vi "Assert No Error.vi"(7 "Status":T1=enum."Failed", 8 "error In":errorcluster, 10 "Assert error":errorcluster, 11 "LUnit Test Case In":refnum<class "LUnit Test Case V2.lvclass">) -> (0 "error out":errorcluster, 3 "LUnit Test Case Out":refnum<class "LUnit Test Case V2.lvclass">)   [LabVIEW 2020, in "LUnit Test Case V2.lvclass"]
doc: "Generates a fail result for the calling test method if the inputs contains an error with status \"True\". A description may be provided to the result."
uses:
  LUnit Test Case V2.lvclass
  Result/Status.ctl
  Result/Type.ctl
  Result/Result.ctl
  LUnit Test Case V2.lvclass/LUnit Test Case V2.ctl
  Result/Result.lvlib
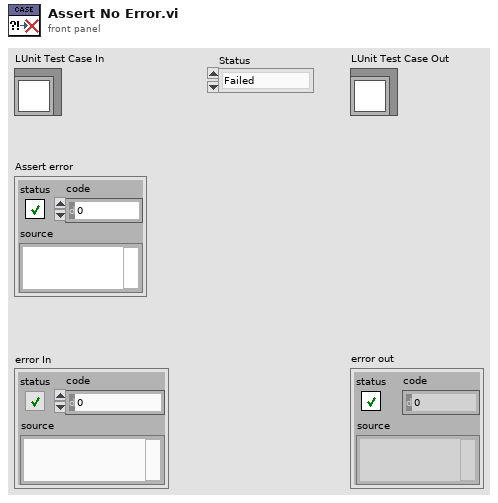
[diagram p1: front panel]
types:
  T1 = typedef "Result.lvlib/Status.ctl" = enum16{"", "Passed", "Failed", "Error", "Skipped", "Setup Error", "Broken", "Teardown Error"}
  T2 = typedef "Result.lvlib/Type.ctl" = enum16{"Method", "Case", "Suite", "Pass", "Fail", "Skip", "Pass if", "Fail if", "Pass if Error", "Fail if Error", "Pass if Equal", "Fail if Equal"}
  T3 = typedef "Result.lvlib/Result.ctl" = cluster{"Name":string, "Message":string, "Description":string, "Status":T1, "Result Type":T2, "Execution Time":dbl}
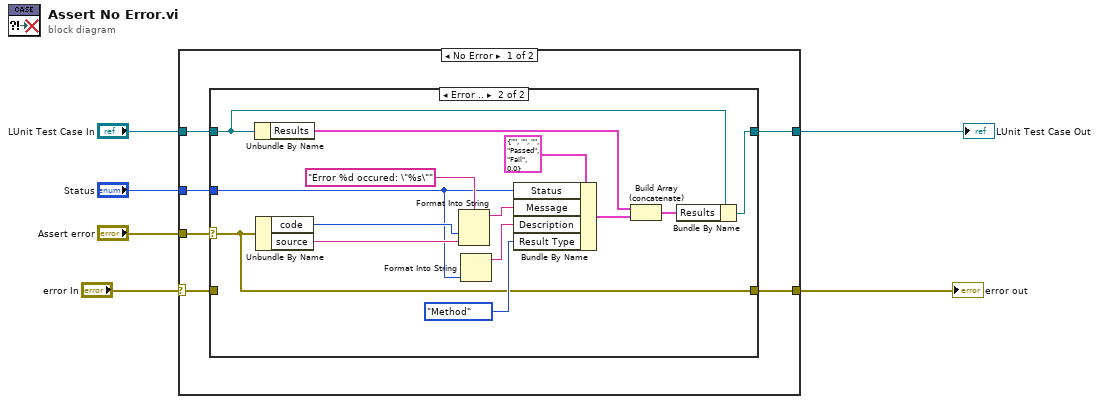
[diagram p0: block diagram]
diagram:
  n1 = case shown="No Error" "error In" {
    selector: "error In" -> [w7 w30]
    tunnel: "Assert error" -> [w12 _]
    tunnel: "LUnit Test Case In" -> [w11 w29]
    tunnel: [w10 w29] -> w4
    tunnel: "Status" -> [w9 _]
    tunnel: [w8 w30] -> w2
    frame No Error {
      n2 = case shown="Error .." w12 {
        selector: w12 -> [_ w15]
        tunnel: w11 -> [w14 w28]
        tunnel: [w14 w27] -> w10
        tunnel: w9 -> [_ w17]
        tunnel: [w13 w15] -> w8
        tunnel: w7 -> [w13 _]
        frame No Error {
        }
        frame Error {
          n3 = Unbundle By Name(w28) -> ("Results"=w21:T3[])
          n4 = Unbundle By Name(w15) -> ("code"=w24:i32, "source"=w23:string)
          n5 = Format Into String(format string="Error %d occured: \"%s\"", w24, w23) -> (resulting string=w26:string)  [unwired: 2 in, 1 out]
          n6 = Format Into String(w17) -> (resulting string=w16:string)  [unwired: 3 in, 1 out]
          n7 = Bundle By Name(cluster=T3 {"Name"="", "Message"="", "Description"="", "Status"=enum."Passed", "Result Type"=enum."Fail", "Execution Time"=0.0} ("Temporary Assertion Result"), "Status"=w17, "Message"=w26, "Description"=w16, "Result Type"=Type."Method") -> (w20:T3)
          n8 = Build Array (concatenate)(w21, w20) -> (w22:T3[])
          n9 = Bundle By Name(cluster=w28, "Results"=w22) -> (w27:refnum<class "LUnit Test Case V2.lvclass">)
        }
      }
    }
    frame Error {
    }
  }
  "error out" <- w2
  "LUnit Test Case Out" <- w4
